vi "SetMenu.vi"(8 "error in (no error)":errorcluster caption="错误输入（无错误）", 10 "菜单引用":refnum<k9>, 11 "TPlot 输入":refnum<class "TPlot.lvclass">) -> (0 "error out":errorcluster caption="错误输出", 3 "TPlot 输出":refnum<class "TPlot.lvclass">)   [LabVIEW 2018, in "DataDisplay.lvlib" / "TPlot.lvclass"]
uses:
  TPlot.lvclass
  TPlot.lvclass/TPlot.ctl
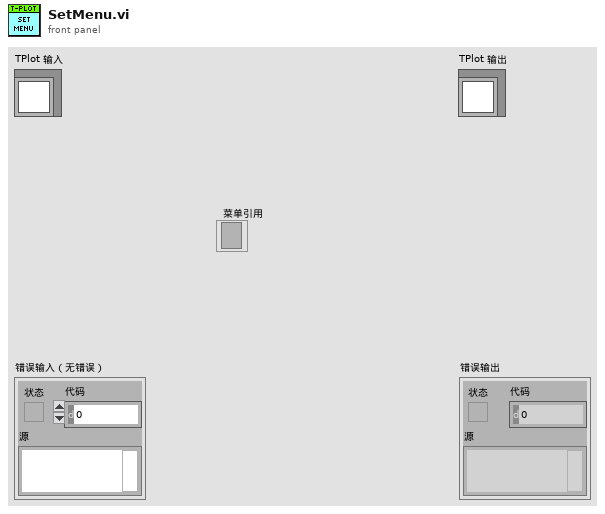
[diagram p1: front panel]
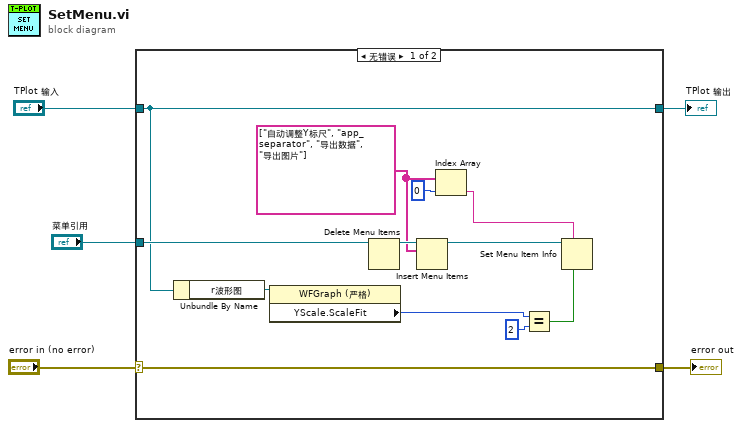
[diagram p0: block diagram]
diagram:
  n1 = case shown="无错误" "error in (no error)" {
    selector: "error in (no error)" -> [w17 w19]
    tunnel: [w17 w19] -> w4
    tunnel: [w13 w18] -> w2
    tunnel: "TPlot 输入" -> [w13 w18]
    tunnel: "菜单引用" -> [w15 _]
    frame No Error {
      w14 = string[] ["自动调整Y标尺", "app_separator", "导出数据", "导出图片"] ("项标识符")
      n2 = Unbundle By Name(w13) -> ("r波形图"=w12:refnum<vi>)
      n3 = property class="WFGraph (严格)"(reference=w12) -> ("YScale.ScaleFit"=w11:u8)  [unwired: 1 in, 2 out]
      n4 = Delete Menu Items(9:w15) -> (3:w16:refnum<k9>)  [unwired: 3 in, 1 out]
      n5 = Insert Menu Items(8:w14, 9:w16) -> (3:w8:refnum<k9>)  [unwired: 4 in, 2 out]
      n6 = Index Array(array=w14, index=0 ("索引")) -> (element=w10:string)
      n7 = Equal?(x=w11, y=u8 2) -> (x = y?=w6:bool)
      n8 = Set Menu Item Info(6:w6, 7:w10, 11:w8) -> ()  [unwired: 4 in, 2 out]
    }
    frame Error {
    }
  }
  "error out" <- w4
  "TPlot 输出" <- w2
